vi "Crop and decimate functional data.vi"(9 "Data in":T1) -> (1 "Data out":T1)   [LabVIEW 2013]
uses:
  xcontrol/Interface VIs/Interface typedefs/Interface-Data array.ctl
  xcontrol/Interface VIs/Interface typedefs/Interface-Data format definition.ctl
  xcontrol/Typedefs/Xctl-XY data type definition.ctl
  xcontrol/Typedefs/Xctrl-ROI type enum.ctl
  xcontrol/Globals/gl_X-Grapher refs.vi
  xcontrol/XGrapher.xctl
panel:
  in  "error in (no error)":errorcluster
  out "out":i32
  out "Nominal number of points shown in the graph":u32=2000
  out "in":i32
  out "# points in selected range":dbl
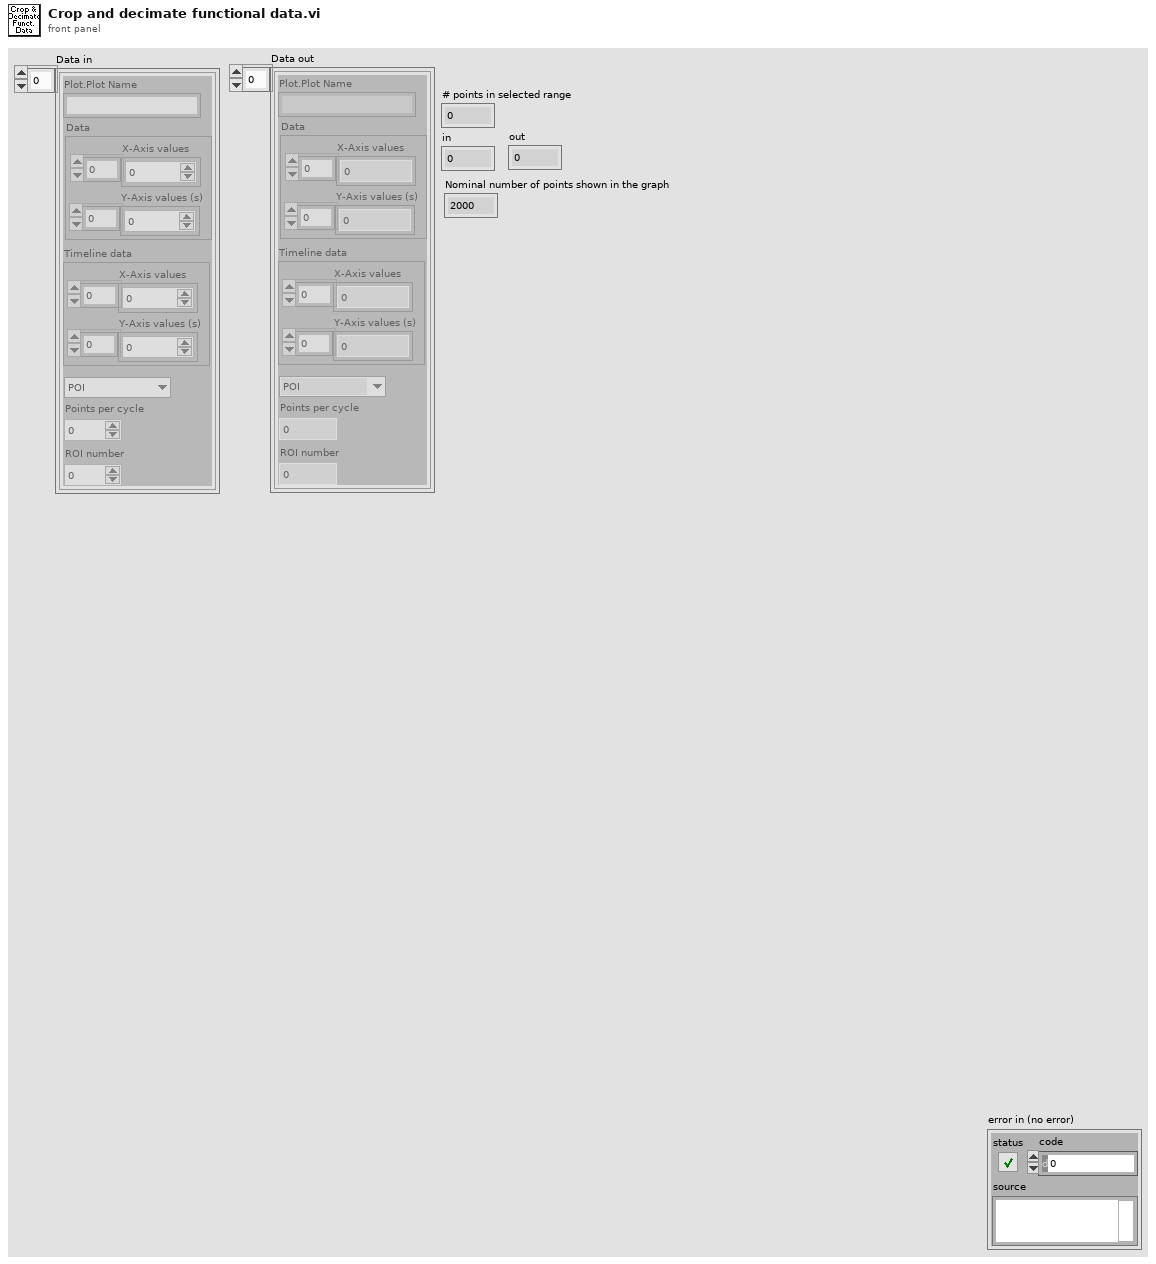
[diagram p1: front panel]
types:
  T1 = typedef "Interface-Data array.ctl" = T2[]
  T2 = typedef "Interface-Data format definition.ctl" = cluster{"Plot.Plot Name":string, "Data":T3, "Timeline data":T3, "Type":T4, "Points per cycle":u16, "ROI number":u16}
  T3 = typedef "XGrapher.xctl/Xctl-XY data type definition.ctl" = cluster{"X-Axis values":sgl[], "Y-Axis values (s)":i32[]}
  T4 = typedef "Xctrl-ROI type enum.ctl" = enum16{"POI", "Mini-scan", "Group"}
  T5 = typedef "XGrapher.xctl/Xctrl-Waveform graph ref.ctl" = refnum<vi>
  T6 = typedef "XGrapher.xctl/Xctrl-Timeline graph ref.ctl" = refnum<vi>
  T7 = typedef "LVRangeTypeDef.ctl" = cluster{"Minimum":dbl, "Maximum":dbl, "Increment":dbl, "Minor Increment":dbl, "Start":dbl}
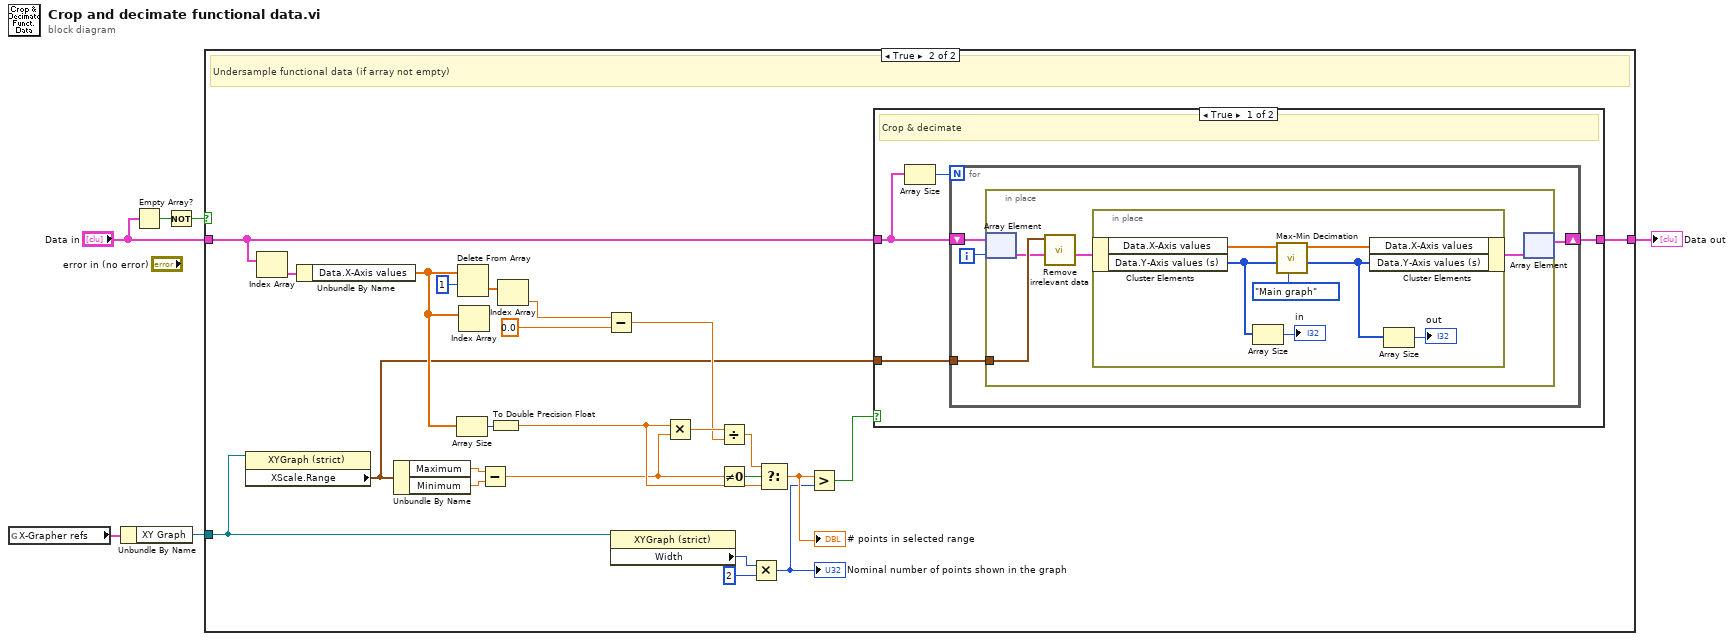
[diagram p0: block diagram]
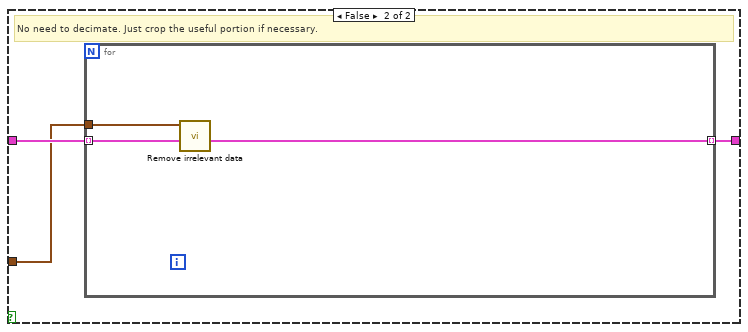
[diagram p3: hidden frame]
diagram:
  n1 = global read "gl_X-Grapher refs.vi" "X-Grapher refs"() -> (w2:cluster{"XY Graph":T5, "Timeline Graph":T6})
  n2 = Unbundle By Name(w2) -> ("XY Graph"=w1:T5)
  n3 = Empty Array?(array="Data in") -> (empty?=w5:bool)
  n4 = Not(x=w5) -> (.not. x?=w4:bool)
  n5 = case shown="True" w4 {
    tunnel: "Data in" -> [w7 w30]
    tunnel: [w7 w31] -> w6
    tunnel: w1 -> [_ w9]
    frame False {
      # "Normalisation turned OFF OR no data array is empty"
    }
    frame True {
      # "Undersample functional data (if array not empty)"
      n6 = property class="XYGraph (strict)"(reference=w9) -> ("XScale.Range"=w8:T7)  [unwired: 1 in, 2 out]
      n7 = Index Array(array=w30) -> (element=w29:T2)  [unwired: 1 in]
      n8 = Unbundle By Name(w29) -> ("Data.X-Axis values"=w22:sgl[])
      n9 = Unbundle By Name(w8) -> ("Maximum"=w27:dbl, "Minimum"=w26:dbl)
      n10 = Array Size(array=w22) -> (size(s)=w25:i32)
      n11 = Delete From Array(array=w22, length=1) -> (deleted portion=w23:sgl[])  [unwired: 1 in, 1 out]
      n12 = Index Array(array=w22) -> ()  [unwired: 1 in, 1 out]
      n13 = Subtract(x=w27, y=w26) -> (x-y=w13:dbl)
      n14 = To Double Precision Float(number=w25) -> (double precision float=w18:dbl)
      n15 = Index Array(array=w23) -> (element=w21:sgl)  [unwired: 1 in]
      n16 = Subtract(x=w21, y=0.0 ("element")) -> (x-y=w14:dbl)
      n17 = property on="Property Node" class="XYGraph (strict)"(reference=w9) -> ("Width"=w11:u32)  [unwired: 1 in, 2 out]
      n18 = Multiply(x=w18, y=w13) -> (x*y=w24:dbl)
      n19 = Divide(x=w24, y=w14) -> (x/y=w19:dbl)
      n20 = Not Equal To 0?(x=w13) -> (x != 0?=w20:bool)
      n21 = Multiply(x=w11, y=u32 2) -> (x*y=w10:u32)
      "Nominal number of points shown in the graph" <- w10
      n22 = Select(t=w19, s=w20, f=w18) -> (s? t:f=w16:dbl)
      "# points in selected range" <- w16
      n23 = Greater?(x=w16, y=w10) -> (0:w17:bool)
      n24 = case shown="True" w17 {
        tunnel: [w35 w53] -> w31
        tunnel: w30 -> [w32 w52]
        tunnel: w8 -> [w34 w51]
        frame True {
          # "Crop & decimate"
          n25 = Array Size(array=w32) -> (size(s)=w33:i32)
          n26 = for {
            N: w33 -> [_]
            tunnel: w34 -> [w39]
            shift-right: [w37] -> w35
            shift-left: w32 -> [w36]
            i -> [w38]
            n27 = in-place {
              in-place-border: w39 -> [w42]
              n28 = in-place-array #1(w36, w38) -> (w41:T2)
              n29 = call "Remove irrelevant data.vi"("Input cluster"=w41, "XGrapher Range"=w42) -> ("output cluster"=w43:T2)  [unwired: 8 in, 1 out]
              n30 = in-place {
                n31 = in-place-cluster #2(w43) -> ("Data.X-Axis values"=w50:sgl[], "Data.Y-Axis values (s)"=w46:i32[])
                n32 = Array Size(array=w46) -> (size(s)=→"in":i32)
                n33 = call "Max-Min Decimation.vi"("Which graph?"=enum16{"Main graph", "Timeline graph"}."Main graph", "Data.Y-Axis values"=w46, "Data.X-Axis values"=w50) -> ("Data.Y-Axis values"=w45:i32[], "Data.X-Axis values"=w49:sgl[])  [unwired: 7 in]
                n34 = in-place-cluster #2("Data.X-Axis values"=w49, "Data.Y-Axis values (s)"=w45) -> (w40:T2)
                n35 = Array Size(array=w45) -> (size(s)=→"out":i32)
              }
              n36 = in-place-array #1(w40) -> (w37:T1)  [unwired: 1 out]
            }
          }
        }
        frame False {
          # "No need to decimate. Just crop the useful portion if necessary."
          n37 = for {
            tunnel: w52 -> [w56] mode=indexing
            tunnel: [w54] -> w53 mode=indexing
            tunnel: w51 -> [w55]
            n38 = call "Remove irrelevant data.vi"("Input cluster"=w56, "XGrapher Range"=w55) -> ("output cluster"=w54:T2)  [unwired: 8 in, 1 out]
          }
        }
      }
    }
  }
  "Data out" <- w6
